vi "Manager Run Main.vi"(8 "error in":errorcluster) -> (0 "error out":errorcluster)   [LabVIEW 2020, in "Manager.lvlib"]
uses:
  Manager.lvlib
  Shared Ressources/raised-error-cluster.ctl
  SubVIs and TypeDefs/Eventing/Event FGV Actions.ctl
  SubVIs and TypeDefs/Manager Runtime Data.ctl
  Shared Ressources/latest-controller-inputs.ctl
  Shared Ressources/Controller-button-pressed-enum.ctl
  Shared Ressources/gamepad-direction-enum.ctl
  Shared Ressources/gui-data-to-display-cluster.ctl
  GUI/GUI.lvlib
  Hardware/Hardware.lvlib
panel:
  in  "raised error":T1={"stop?"=FALSE, "cause"="Error"}
  out "Event Iterations":i32
  # "Event Handler: Run Main VI"
  # "Icon Attribution\n<div>Icons made by <a href=\"https://www.freepik.com \" title=\"Freepik\">Freepik</a> from <a href=\"https://www.flaticon.com/ \" title=\"Flaticon\">www.flaticon.com</a></div>"
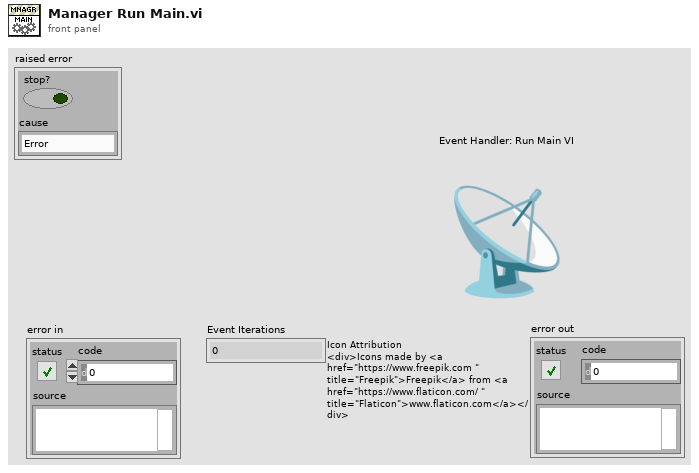
[diagram p1: front panel]
types:
  T1 = typedef "raised-error-cluster.ctl" = cluster{"stop?":bool, "cause":string}
  T2 = typedef "Controller-button-pressed-enum.ctl" = enum16{"button 1", "button 2", "button 3", "button 4", "button 5", "button 6", "button 7", "button 8", "button 9", "button 10", "button 11", "button 12", "button 13", "button 14"}
  T3 = typedef "Manager.lvlib/Manager Runtime Data.ctl" = cluster{"ui tempo":dbl, "latest controller inputs":T4, "information":string}
  T4 = typedef "latest-controller-inputs.ctl" = cluster{"Controller button pressed enum":T2, "gamepad direction":T5}
  T5 = typedef "gamepad-direction-enum.ctl" = enum16{"Up Arrow", "Right Arrow", "Down Arrow", "Left Arrow"}
  T6 = typedef "Manager.lvlib/Event FGV Actions.ctl" = enum16{"Get", "Create", "Destroy"}
  T7 = typedef "gui-data-to-display-cluster.ctl" = cluster{"latest controller inputs":T4, "information":string}
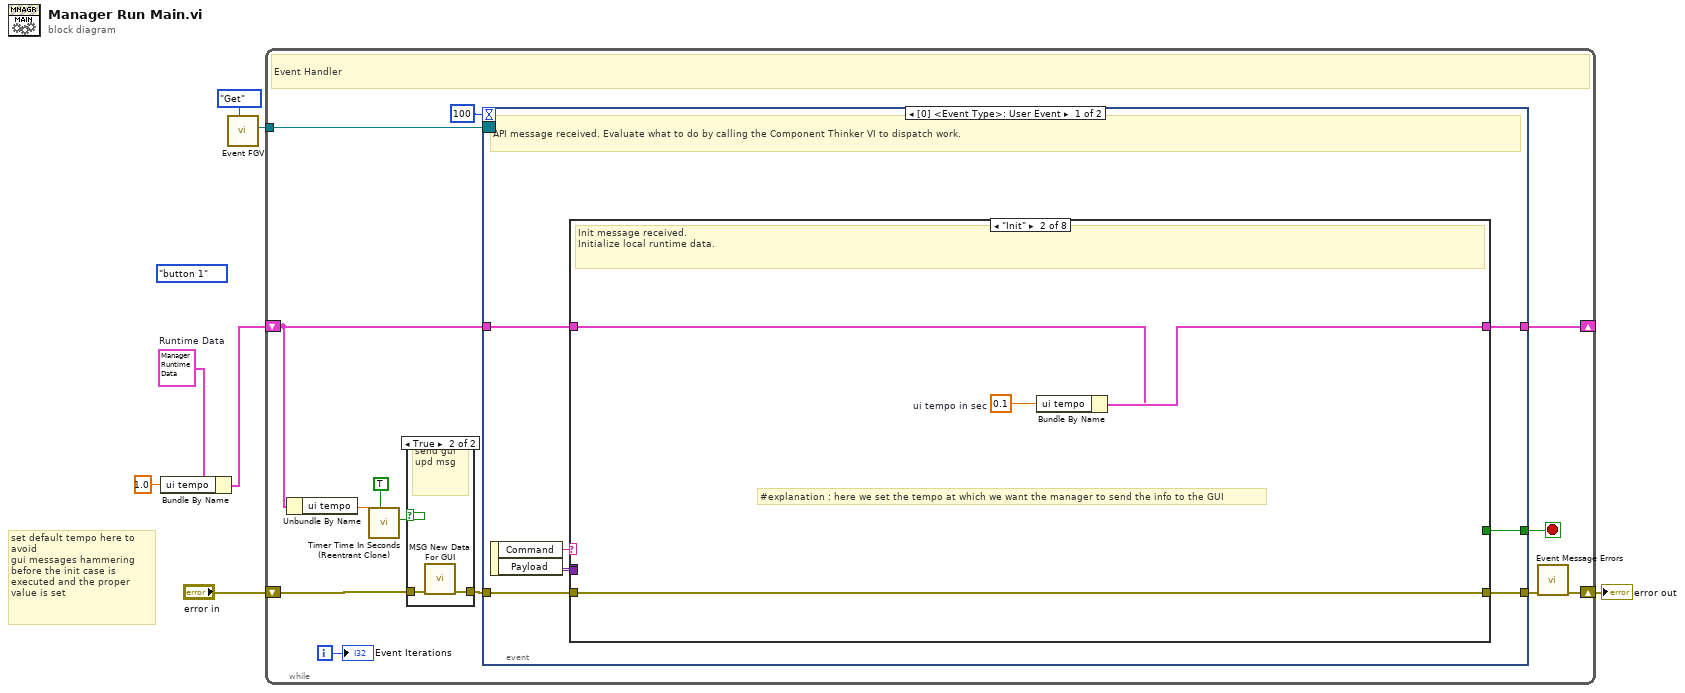
[diagram p0: block diagram]
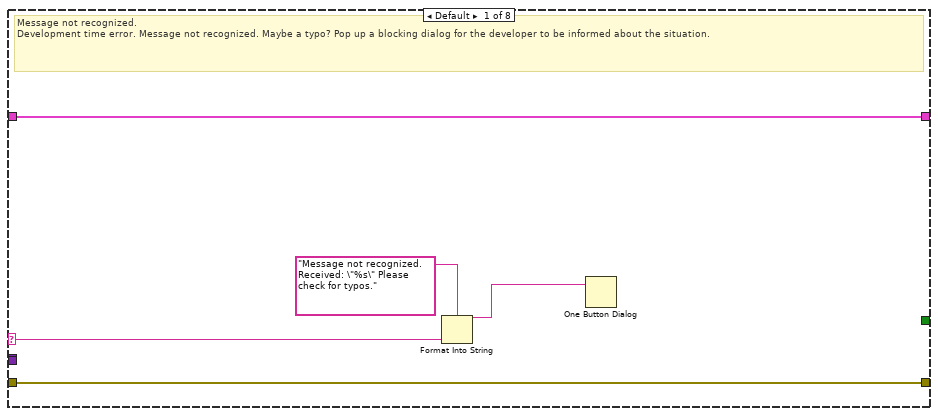
[diagram p3: hidden frame]
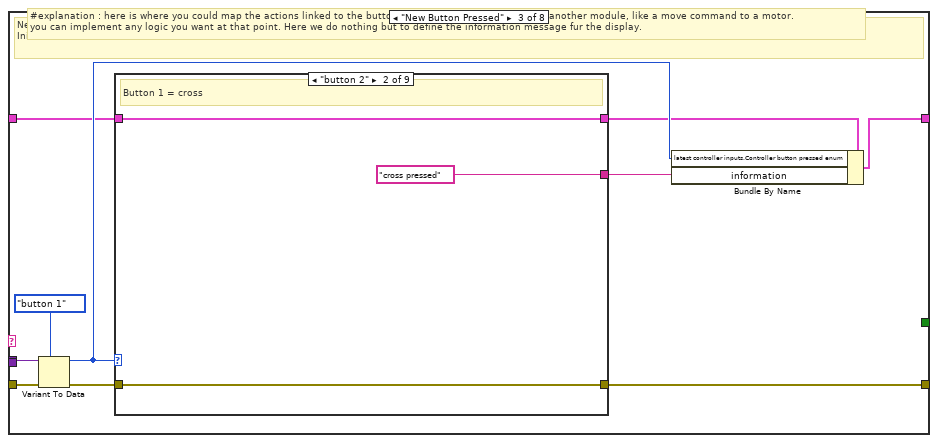
[diagram p4: hidden frame]
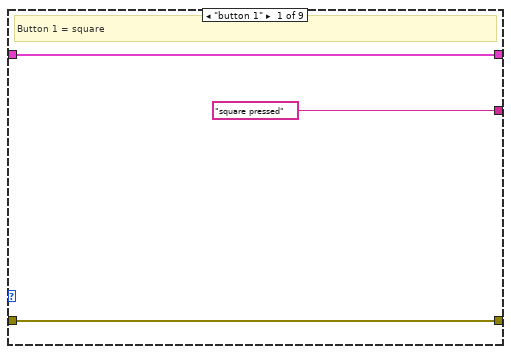
[diagram p5: hidden frame]
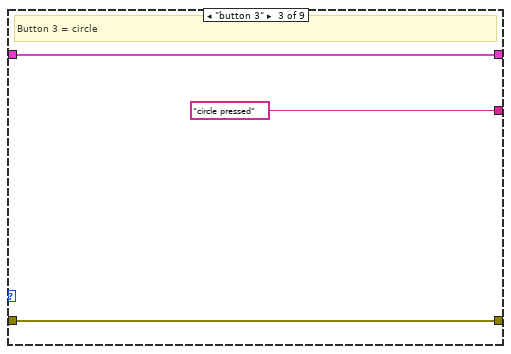
[diagram p6: hidden frame]
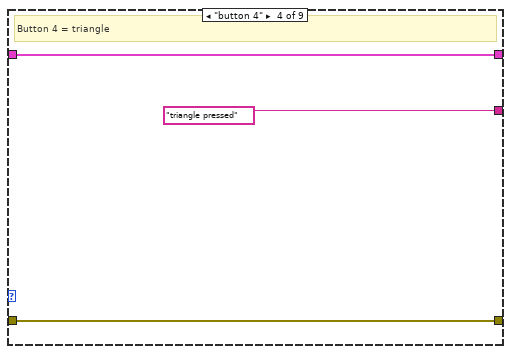
[diagram p7: hidden frame]
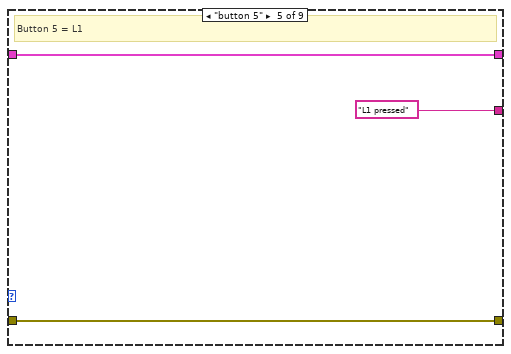
[diagram p8: hidden frame]
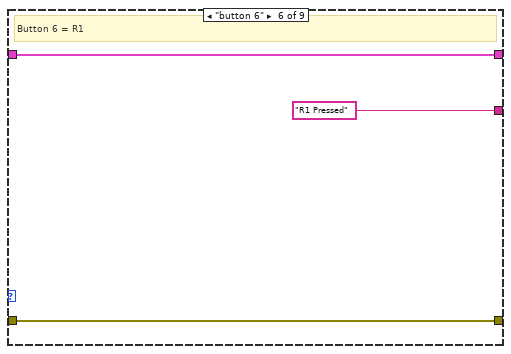
[diagram p9: hidden frame]
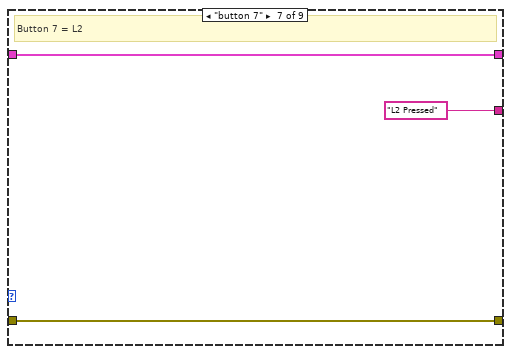
[diagram p10: hidden frame]
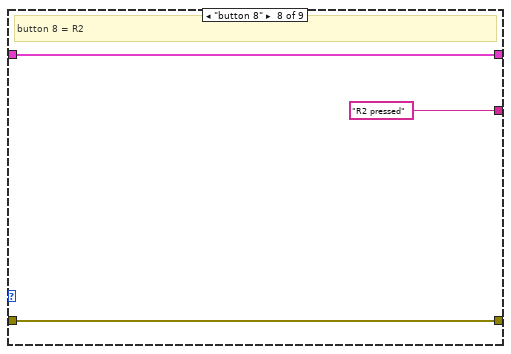
[diagram p11: hidden frame]
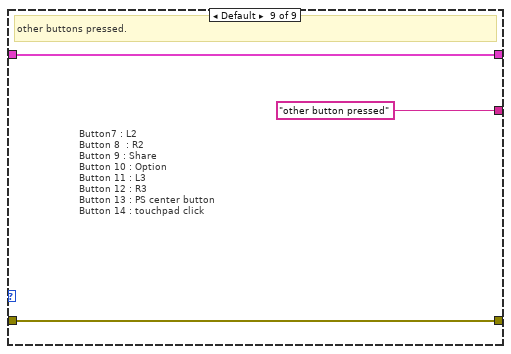
[diagram p12: hidden frame]
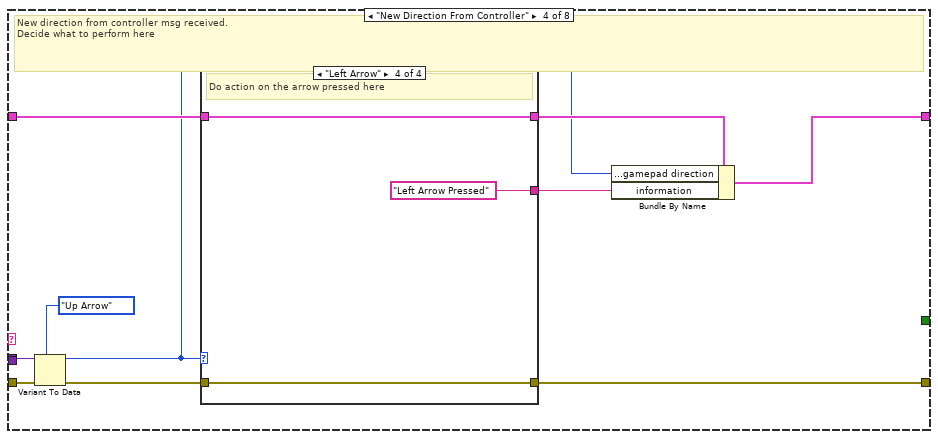
[diagram p13: hidden frame]
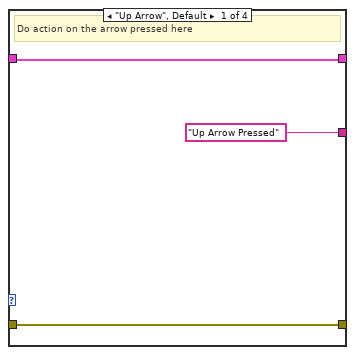
[diagram p14: hidden frame]
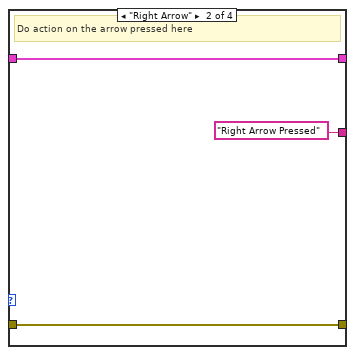
[diagram p15: hidden frame]
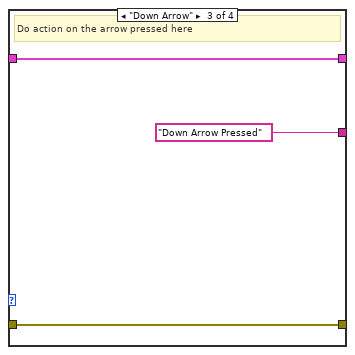
[diagram p16: hidden frame]
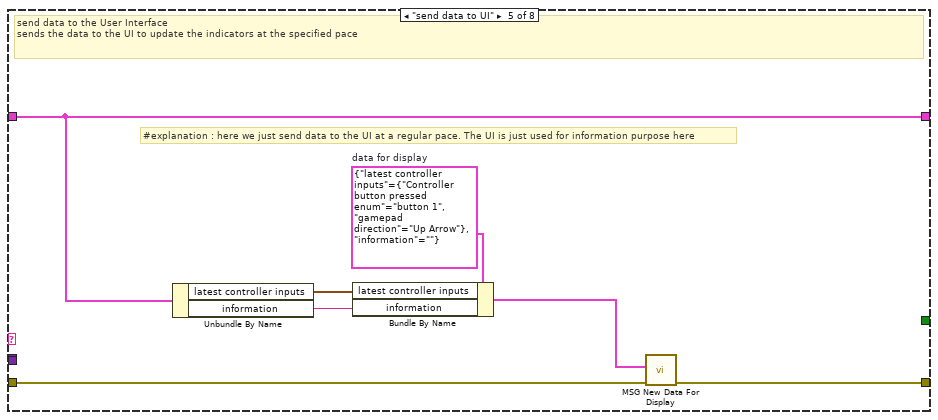
[diagram p17: hidden frame]
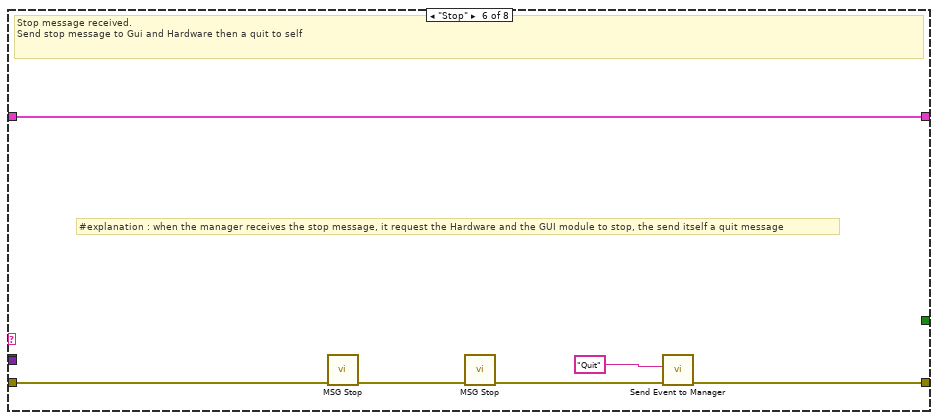
[diagram p18: hidden frame]
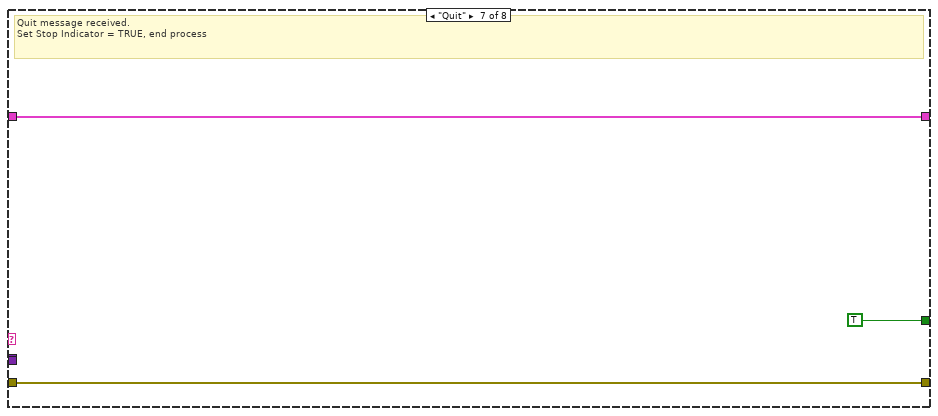
[diagram p19: hidden frame]
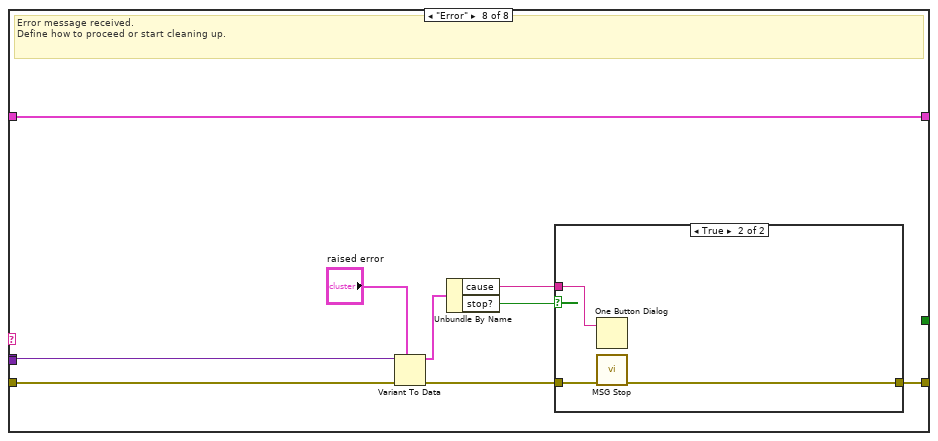
[diagram p20: hidden frame]
diagram:
  (unwired) Controller-button-pressed-enum."button 1" ("Controller button pressed enum")
  w2 = T3 {"ui tempo"=50.0, "latest controller inputs"={"Controller button pressed enum"=enum."button 1", "gamepad direction"=enum."Up Arrow"}, "information"=""}  # Runtime Data
  # "set default tempo here to avoid\ngui messages hammering before the init case is executed and the proper value is set"
  n1 = Bundle By Name(cluster=w2, "ui tempo"=1.0) -> (w1:T3)
  n2 = call "Event FGV.vi"("Event FGV Actions"=Event_FGV_Actions."Get") -> ("Event Registration Refnum"=w4:refnum<event-registration>)  [unwired: 8 in, 2 out]
  n3 = while {
    shift-right: [w17] -> w6
    shift-left: "error in" -> [w8]
    tunnel: w4 -> [w20]
    shift-right: [w16] -> _
    shift-left: w1 -> [w13]
    i -> [w19]
    stop <- w15 stop-if-true
    # "Event Handler"
    n4 = Unbundle By Name(w13) -> ("ui tempo"=w12:dbl)
    n5 = call "Timer Time In Seconds (Reentrant Clone).vi"("Auto Reset?"=TRUE, "Elapsed Time Target [s]"=w12) -> ("Time has Elapsed"=w10:bool)  [unwired: 8 in, 1 out]
    n6 = case shown="True" w10 {
      tunnel: [w21 w22] -> w9
      tunnel: w8 -> [w21 w23]
      frame False {
      }
      frame True {
        # "send gui upd msg"
        n7 = call "MSG New Data For GUI.vi"("error in"=w23) -> ("error out"=w22:errorcluster)  [unwired: 10 in]
      }
    }
    n8 = event shown="[0] <Event Type>: User Event" {
      selector: w20 -> [_ _]
      dyn-events: _ -> [_ _]
      timeout: 100 -> [_ _]
      tunnel: [w24 w137] -> w18
      tunnel: w9 -> [w29 w137]
      tunnel: [w27 w136] -> w16
      tunnel: w13 -> [w30 w136]
      tunnel: [w26 _] -> w15
      event User Event {
        # "API message received. Evaluate what to do by calling the Component Thinker VI to dispatch work."
        n9 = event-data() -> ("Command"=w28:string, "Payload"=w25:variant)  [unwired: 1 in]
        n10 = case shown="\"Init\"" w28 {
          selector: w28 -> [w34 _ _ _ _ _ _ _]
          tunnel: w29 -> [w32 w36 w48 w86 w105 w111 w113 w123]
          tunnel: w25 -> [_ _ w49 w78 _ _ _ w122]
          tunnel: [_ _ _ _ _ _ TRUE _] -> w26
          tunnel: w30 -> [w31 w38 w43 w83 w104 w110 w112 w115]
          tunnel: [w31 w39 w46 w84 w104 w110 w112 w115] -> w27
          tunnel: w25 -> [_ _ _ _ _ _ _ _]
          tunnel: [w32 w36 w40 w80 w103 w107 w113 w116] -> w24
          frame Default {
            # "Message not recognized.\nDevelopment time error. Message not recognized. Maybe a typo? Pop up a blocking dialog for the developer to be informed about the situation."
            n11 = Format Into String(format string="Message not recognized. Received: \"%s\" Please check for typos." ("message"), w34) -> (resulting string=w33:string)  [unwired: 2 in, 1 out]
            n12 = One Button Dialog(message=w33) -> ()  [unwired: 1 in, 1 out]
          }
          frame "Init" {
            w37 = 0.1  # ui tempo in sec
            # "#explanation : here we set the tempo at which we want the manager to send the info to the GUI"
            # "Init message received.\nInitialize local runtime data."
            n13 = Bundle By Name(cluster=w38, "ui tempo"=w37) -> (w39:T3)
          }
          frame "New Button Pressed" {
            # "#explanation : here is where you could map the actions linked to the buttons. typically, send a message to another module, like a move command to a motor.\nyou can implement any logic you want at that point. Here we do nothing but to define the information message fur the display."
            # "New button Pressed msg received.\nInitialize local runtime data."
            n14 = Variant To Data(error in=w48, type=Controller-button-pressed-enum."button 1" ("Controller button pressed enum"), Variant=w49) -> (data=w45:T2, error out=w41:errorcluster)
            n15 = case shown="\"button 2\"" w45 {
              tunnel: w43 -> [w50 w53 w56 w59 w62 w65 w68 w71 w76]
              tunnel: ["square pressed" "cross pressed" "circle pressed" "triangle pressed" "L1 pressed" "R1 Pressed" "L2 Pressed" "R2 pressed" "other button pressed"] -> w42
              tunnel: [w50 w53 w56 w59 w62 w65 w68 w71 w76] -> w44
              tunnel: w41 -> [w51 w54 w57 w60 w63 w66 w70 w73 w74]
              tunnel: [w51 w54 w57 w60 w63 w66 w70 w73 w74] -> w40
              frame "button 1" {
                # "Button 1 = square"
              }
              frame "button 2" {
                # "Button 1 = cross"
              }
              frame "button 3" {
                # "Button 3 = circle"
              }
              frame "button 4" {
                # "Button 4 = triangle"
              }
              frame "button 5" {
                # "Button 5 = L1"
              }
              frame "button 6" {
                # "Button 6 = R1"
              }
              frame "button 7" {
                # "Button 7 = L2"
              }
              frame "button 8" {
                # "button 8 = R2"
              }
              frame Default {
                # "Button7 : L2\nButton 8  : R2\nButton 9 : Share\nButton 10 : Option\nButton 11 : L3\nButton 12 : R3\nButton 13 : PS center button\nButton 14 : touchpad click"
                # "other buttons pressed."
              }
            }
            n16 = Bundle By Name(cluster=w44, "latest controller inputs.Controller button pressed enum"=w45, "information"=w42) -> (w46:T3)
          }
          frame "New Direction From Controller" {
            # "New direction from controller msg received.\nDecide what to perform here"
            n17 = Variant To Data(error in=w86, type=gamepad-direction-enum."Up Arrow" ("latest controller inputs.gamepad direction"), Variant=w78) -> (data=w77:T5, error out=w79:errorcluster)
            n18 = case shown="\"Left Arrow\"" w77 {
              tunnel: [w88 w92 w95 w97] -> w82
              tunnel: w83 -> [w88 w92 w95 w97]
              tunnel: ["Up Arrow Pressed" "Right Arrow Pressed" "Down Arrow Pressed" "Left Arrow Pressed"] -> w81
              tunnel: [w87 w90 w93 w96] -> w80
              tunnel: w79 -> [w87 w90 w93 w96]
              frame "Up Arrow", Default {
                # "Do action on the arrow pressed here"
              }
              frame "Right Arrow" {
                # "Do action on the arrow pressed here"
              }
              frame "Down Arrow" {
                # "Do action on the arrow pressed here"
              }
              frame "Left Arrow" {
                # "Do action on the arrow pressed here"
              }
            }
            n19 = Bundle By Name(cluster=w82, "latest controller inputs.gamepad direction"=w77, "information"=w81) -> (w84:T3)
          }
          frame "send data to UI" {
            w102 = T7 {"latest controller inputs"={"Controller button pressed enum"=enum."button 1", "gamepad direction"=enum."Up Arrow"}, "information"=""}  # data for display
            # "#explanation : here we just send data to the UI at a regular pace. The UI is just used for information purpose here"
            # "send data to the User Interface\nsends the data to the UI to update the indicators at the specified pace"
            n20 = Unbundle By Name(w104) -> ("latest controller inputs"=w100:T4, "information"=w99:string)
            n21 = Bundle By Name(cluster=w102, "latest controller inputs"=w100, "information"=w99) -> (w101:T7)
            n22 = call "MSG New Data For Display.vi"("error in"=w105, "Payload"=w101) -> ("error out"=w103:errorcluster)  [unwired: 9 in]
          }
          frame "Stop" {
            # "#explanation : when the manager receives the stop message, it request the Hardware and the GUI module to stop, the send itself a quit message"
            # "Stop message received.\nSend stop message to Gui and Hardware then a quit to self"
            n23 = call "MSG Stop.vi"("error in"=w111) -> ("error out"=w109:errorcluster)  [unwired: 10 in]
            n24 = call "MSG Stop.vi"("error in"=w109) -> ("error out"=w108:errorcluster)  [unwired: 10 in]
            n25 = call "Send Event to Manager.vi"("error in"=w108, "Command"="Quit") -> ("error out"=w107:errorcluster)  [unwired: 9 in]
          }
          frame "Quit" {
            # "Quit message received.\nSet Stop Indicator = TRUE, end process"
          }
          frame "Error" {
            # "Error message received.\nDefine how to proceed or start cleaning up."
            n26 = Variant To Data(error in=w123, type="raised error", Variant=w122) -> (data=w120:T1, error out=w118:errorcluster)
            n27 = Unbundle By Name(w120) -> ("cause"=w117:string, "stop?"=w119:bool)
            n28 = case shown="True" w119 {
              tunnel: [w129 w134] -> w116
              tunnel: w118 -> [_ w135]
              tunnel: w117 -> [w128 w133]
              frame False {
                n29 = Concatenate Strings(w128, "\nDo you want to continue using the application?" ("T button name (\"OK\")")) -> (w126:string)
                n30 = Two Button Dialog(message=w126, 1:"No, stop" ("F button name (\"Cancel\")"), 2:"Yes, continue" ("T button name (\"OK\")")) -> (T button?=w130:bool)
                n31 = case shown="False" w130 {
                  tunnel: [w131 errorcluster {"status"=FALSE, "code"=0, "source"=""} ("error out")] -> w129
                  frame False {
                    n32 = call "MSG Stop.vi"() -> ("error out"=w131:errorcluster)  [unwired: 11 in]
                  }
                  frame True {
                  }
                }
              }
              frame True {
                n33 = One Button Dialog(message=w133) -> ()  [unwired: 1 in, 1 out]
                n34 = call "MSG Stop.vi"("error in"=w135) -> ("error out"=w134:errorcluster)  [unwired: 10 in]
              }
            }
          }
        }
      }
      event Timeout {
        # "#CodeOptional: Argument for specifying a timeout: We want the application to remain responsive. The timeout case should only hold code to be executed in this exceptional state. Think 'timeout-warning-error' as increasing levels of escalation severity. A timeout could occur regularly but it doesn't have to. If the event structure receives messages faster than the specified timeout, this case will never be executed."
        n35 = event-data() -> ()  [unwired: 1 in, 3 out]
      }
    }
    n36 = call "Event Message Errors.vi"("error in"=w18) -> ("error out"=w17:errorcluster)  [unwired: 10 in]
    "Event Iterations" <- w19
  }
  "error out" <- w6
